vi "generate_circle_plan.vi"(0 "Radius":dbl, 1 "Lead-in degrees":dbl=45.0, 2 "Number segments":i32, 3 "error in (no error)":errorcluster, 4 "Lead-out degrees":dbl=45.0) -> (6 "Plan":string, 7 "error out":errorcluster)   [LabVIEW 2020]
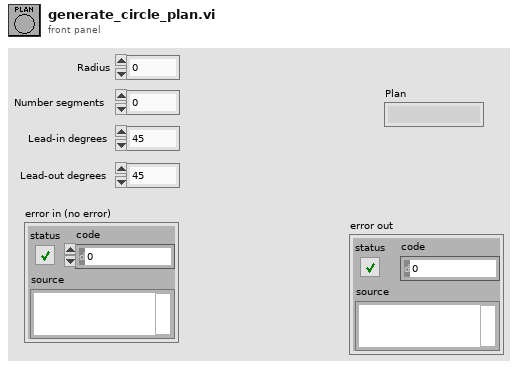
[diagram p1: front panel]
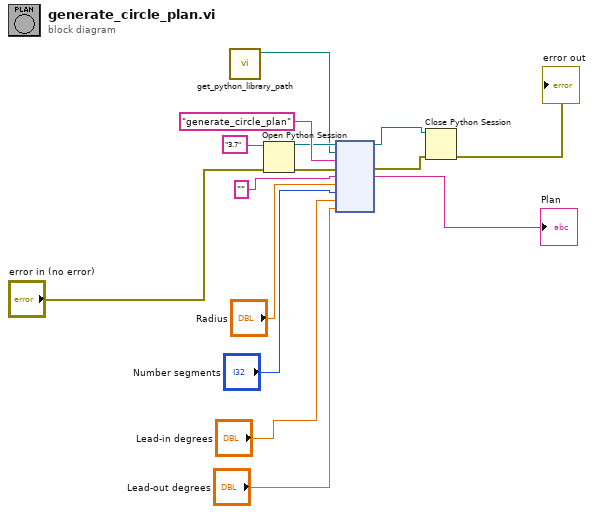
[diagram p0: block diagram]
diagram:
  n1 = call "get_python_library_path.vi"() -> ("Python library path"=w5:path)  [unwired: 11 in]
  n2 = Open Python Session(python version="3.7" ("Python version"), 3:"error in (no error)") -> (session out=w7:refnum<k35>, error out=w9:errorcluster)  [unwired: 1 in]
  n3 = node(w7, w5, "generate_circle_plan" ("function name"), w9, "" ("Python version"), "Radius", "Number segments", "Lead-in degrees", "Lead-out degrees") -> (w14:refnum<k35>, w15:errorcluster, →"Plan":string)  [unwired: 4 in, 2 out]
  n4 = Close Python Session(session in=w14, error in=w15) -> (11:→"error out":errorcluster)
